vi "GetGraphTypeInfo.vi"(0 "reference in":refnum<class "DqmhModuleDiagramGraph.lvclass">, 5 "error in (no error)":errorcluster) -> (14 "reference out":refnum<class "DqmhModuleDiagramGraph.lvclass">, 15 "GraphTypeName":string, 16 "NodeTypes":refnum<class "AbstractNode.lvclass">[](array[class]), 17 "EdgeTypes":refnum<class "AbstractEdge.lvclass">[](array[class]), 18 "GraphTypeUserName":string, 19 "error out":errorcluster)   [LabVIEW 2014, in "DqmhModuleDiagramGraph.lvclass"]
uses:
  <resource>/Framework/Providers/Open_GDS/UML/DqmhModuleDiagramGraph_class/DqmhModuleDiagramGraph.lvclass
  <resource>/Framework/Providers/Open_GDS/UML/AbstractNode_class/AbstractNode.lvclass
  <resource>/Framework/Providers/Open_GDS/UML/AbstractEdge_class/AbstractEdge.lvclass
  <resource>/Framework/Providers/Open_GDS/UML/DQMHModuleNode_class/DQMHModuleNode.lvclass
  <resource>/Framework/Providers/Open_GDS/UML/NoteNode_class/NoteNode.lvclass
  <resource>/Framework/Providers/Open_GDS/UML/ClassRelationshipEdge_class/ClassRelationshipEdge.lvclass
  <resource>/Framework/Providers/Open_GDS/UML/NoteEdge_class/NoteEdge.lvclass
  <resource>/Framework/Providers/Open_GDS/UML/VINode_class/VINode.lvclass
  <resource>/Framework/Providers/Open_GDS/UML/Graph_class/Graph.lvclass
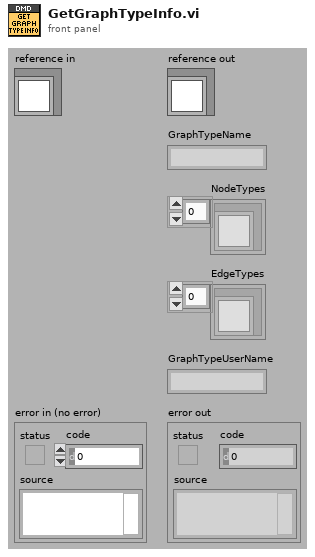
[diagram p1: front panel]
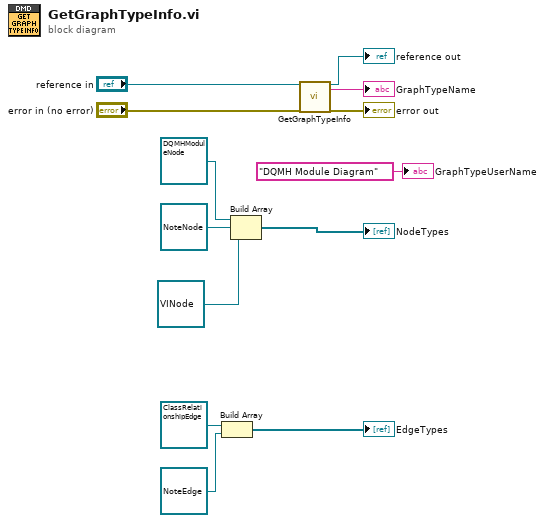
[diagram p0: block diagram]
diagram:
  n1 = Build Array(refnum<class "ClassRelationshipEdge.lvclass"> refnum ("ClassRelationshipEdge.lvclass"), refnum<class "NoteEdge.lvclass"> refnum ("NoteEdge.lvclass")) -> (→"EdgeTypes":refnum<class "GeneralPathEdge.lvclass">[])
  n2 = Build Array(refnum<class "DQMHModuleNode.lvclass"> refnum ("DQMHModuleNode"), refnum<class "NoteNode.lvclass"> refnum ("NoteNode.lvclass"), refnum<class "VINode.lvclass"> refnum ("VINode")) -> (→"NodeTypes":refnum<class "RectangularNode.lvclass">[])
  n3 = call-parent "GetGraphTypeInfo.vi"("reference in"="reference in", "error in (no error)"="error in (no error)") -> ("reference out"=→"reference out":refnum<class "DqmhModuleDiagramGraph.lvclass">, "GraphTypeName"=→"GraphTypeName":string, "error out"=→"error out":errorcluster)  [unwired: 12 in, 3 out]
  "GraphTypeUserName" <- "DQMH Module Diagram" ("GraphTypeUserName")
